vi "Profinet DCP Parsing.vi"(11 "Data in":string="\u0000\f)ÒîD\u0000\u001b\u001bI÷éˆ’þÿ\u0005\u0001\u0000\u0000\u0001k\u0000\u0000\u0000d\u0002\u0005\u0000\u001e\u0000\u0000\u0001\u0001\u0001\u0002\u0002\u0001\u0002\u0002\u0002\u0003\u0002\u0004\u0002\u0005\u0003=\u0005\u0001\u0005\u0002\u0005\u0003\u0005\u0004\u0005\u0005ÿÿ\u0002\u0001\u0000\u000b\u0000\u0000S7-400 CP\u0000\u0002\u0002\u0000\t\u0000\u0000pn-io-1\u0000\u0002\u0003\u0000\u0006\u0000\u0000\u0000*\u0002\u0001\u0002\u0004\u0000\u0004\u0000\u0000\u0002\u0000\u0001\u0002\u0000\u000e\u0000\u0001À¨dVÿÿÿ\u0000\u0000\u0000\u0000\u0000") -> (2 "PROFINET DCP Response":bool, 3 "Profinet Ident":T1)   [LabVIEW 2017]
uses:
  TypeDefs/control_packet_header_ethernet 2.ctl
  TypeDefs/Profinet Ident.ctl
panel:
  out "Device Role":u8[](array[numeric])
  out "Device ID":u8[](array[numeric])
  out "Device/Device Options":u8[](array[numeric])
  out "ethernet header":T2 {"Service ID and Type" format="%04x"; "Frame ID" format="%04x"; "destination MAC address"."?" format="%02x"; "destination MAC address"."?" format="%02x"; "destination MAC address"."?" format="%02x"; "destination MAC address"."?" format="%02x"; "destination MAC address"."?" format="%02x"; "destination MAC address"."?" format="%02x"; "source MAC address"."?" format="%02x"; "source MAC address"."?" format="%02x"; "source MAC address"."?" format="%02x"; "source MAC address"."?" format="%02x"; "source MAC address"."?" format="%02x"; "source MAC address"."?" format="%02x"; "length / type" format="%04x"}
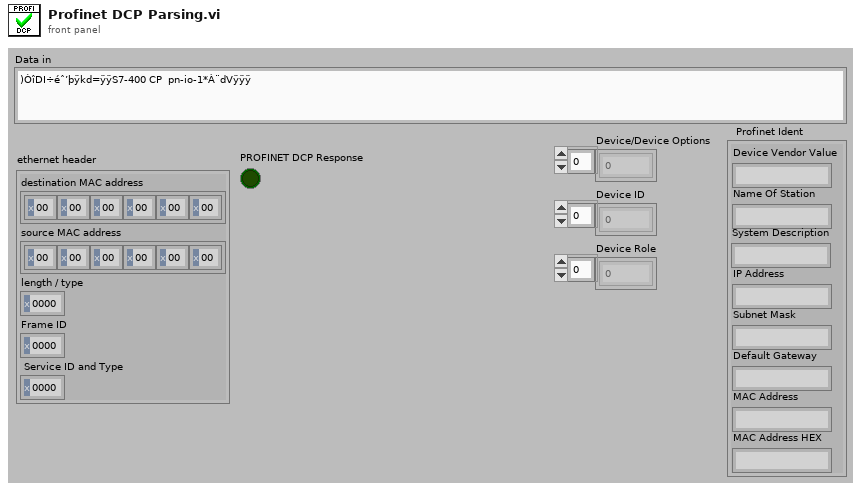
[diagram p1: front panel]
types:
  T1 = typedef "Profinet Ident.ctl" = cluster{"Device Vendor Value":string, "Name Of Station":string, "IP Address":string, "Subnet Mask":string, "Default Gateway":string, "MAC Address":string, "MAC Address HEX":string, "System Description ":string}
  T2 = typedef "control_packet_header_ethernet 2.ctl" = cluster{"destination MAC address":cluster{u8, u8, u8, u8, u8, u8}, "source MAC address":cluster{u8, u8, u8, u8, u8, u8}, "length / type":u16, "Frame ID":u16, " Service ID and Type":u16}
  T3 = enum16{"Device Type", "Device Vendor", "Name of Station", "Device ID", "Device Role", "IP Block", "Profinet Ident Values"}
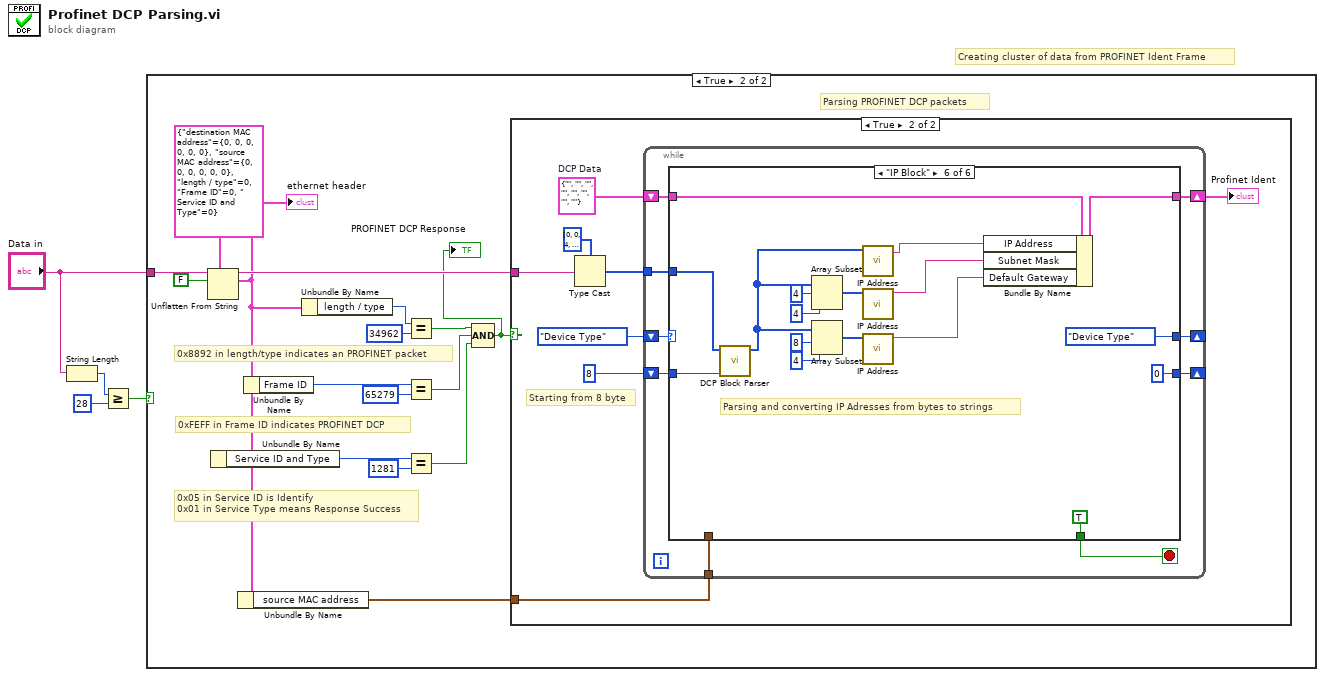
[diagram p0: block diagram]
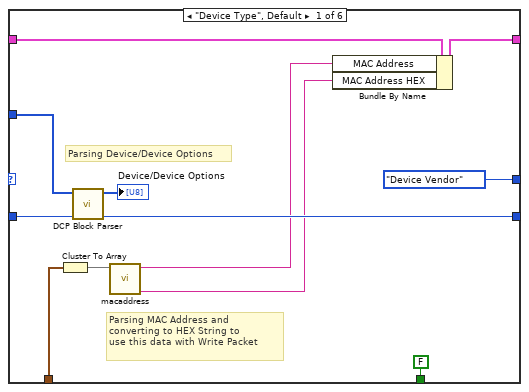
[diagram p4: hidden frame]
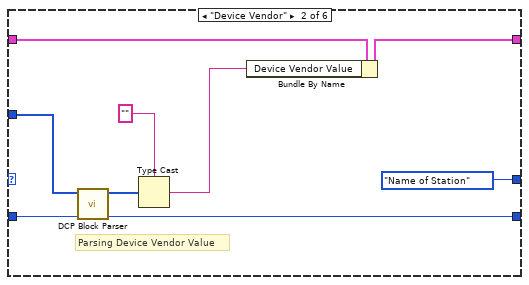
[diagram p5: hidden frame]
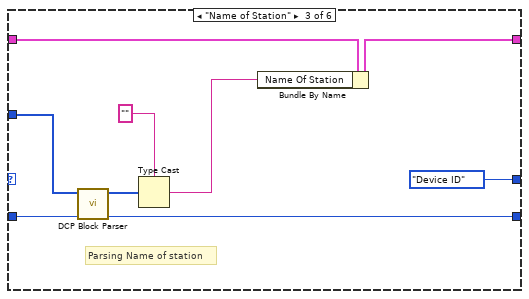
[diagram p6: hidden frame]
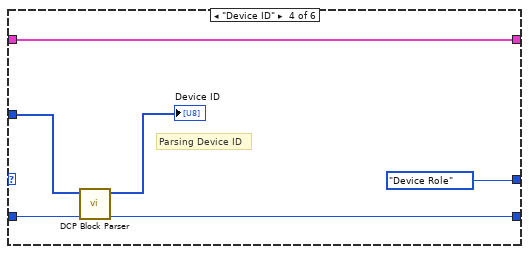
[diagram p7: hidden frame]
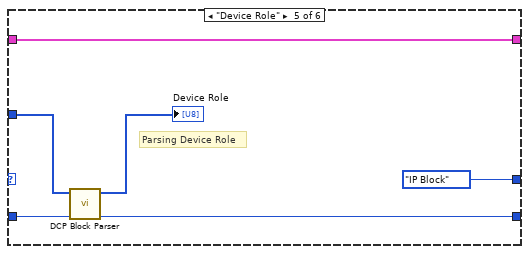
[diagram p8: hidden frame]
diagram:
  # "Creating cluster of data from PROFINET Ident Frame"
  n1 = String Length(string="Data in") -> (length=w3:i32)
  n2 = Greater Or Equal?(x=w3, y=28) -> (x >= y?=w1:bool)
  n3 = case shown="True" w1 {
    tunnel: "Data in" -> [_ w15]
    frame False {
    }
    frame True {
      # "0x05 in Service ID is Identify\n0x01 in Service Type means Response Success"
      # "0xFEFF in Frame ID indicates PROFINET DCP"
      # "Parsing PROFINET DCP packets"
      # "0x8892 in length/type indicates an PROFINET packet"
      n4 = Unflatten From String(type=T2 {"destination MAC address"={0, 0, 0, 0, 0, 0}, "source MAC address"={0, 0, 0, 0, 0, 0}, "length / type"=0, "Frame ID"=0, " Service ID and Type"=0} ("ethernet header"), binary string=w15, data includes array or string size? (T)=FALSE) -> (rest of the binary string=w16:string, value=w13:T2)  [unwired: 2 in, 1 out]
      "ethernet header" <- w13
      n5 = Unbundle By Name(w13) -> ("Service ID and Type"=w7:u16)
      n6 = Unbundle By Name(w13) -> ("source MAC address"=w14:cluster{u8, u8, u8, u8, u8, u8})
      n7 = Unbundle By Name(w13) -> ("Frame ID"=w12:u16)
      n8 = Unbundle By Name(w13) -> ("length / type"=w18:u16)
      n9 = Equal?(x=w18, y=u16 34962) -> (x = y?=w10:bool)
      n10 = Equal?(x=w12, y=u16 65279) -> (x = y?=w9:bool)
      n11 = Equal?(x=w7, y=u16 1281) -> (x = y?=w6:bool)
      n12 = Compound Arithmetic op=AND(w10, w9, w6) -> (w5:bool)
      "PROFINET DCP Response" <- w5
      n13 = case shown="True" w5 {
        tunnel: w16 -> [_ w28]
        tunnel: w14 -> [_ w27]
        frame False {
        }
        frame True {
          w22 = T1 {"Device Vendor Value"="", "Name Of Station"="", "IP Address"="", "Subnet Mask"="", "Default Gateway"="", "MAC Address"="", "MAC Address HEX"="", "System Description "=""}  # DCP Data
          # "Starting from 8 byte"
          n14 = Type Cast(type=u8[] [0, 0, 4, 0, 1, 0, 1, 0, 0, 0, 0, 0, 0, 0, 0, 0, 0, 0, 0, 0, 0, 0, 0, 0, 1, 0, 0, 0] ("Byte Array"), x=w28) -> (*(type *) &x=w25:u8[])
          n15 = while {
            tunnel: w25 -> [w37]
            shift-right: [w34] -> _
            shift-left: T3."Device Type" ("Enum") -> [w36]
            shift-right: [w33] -> _
            shift-left: 8 ("index") -> [w35]
            tunnel: w27 -> [w32]
            shift-right: [w30] -> w21
            shift-left: w22 -> [w29]
            stop <- w31 stop-if-true
            n16 = case shown="\"IP Block\"" w36 {
              tunnel: w37 -> [w49 w58 w67 w73 w79 w96]
              tunnel: w35 -> [w47 w57 w66 w71 w77 w95]
              tunnel: [T3."Device Vendor" ("Enum") T3."Name of Station" ("Enum") T3."Device ID" ("Enum") T3."Device Role" ("Enum") T3."IP Block" ("Enum") T3."Device Type" ("Enum")] -> w34
              tunnel: [w46 w56 w65 w70 w76 0 ("Block Last Byte")] -> w33
              tunnel: w32 -> [w44 _ _ _ _ _]
              tunnel: [FALSE _ _ _ _ TRUE] -> w31
              tunnel: w29 -> [w40 w52 w61 w68 w74 w86]
              tunnel: [w41 w51 w60 w68 w74 w85] -> w30
              frame "Device Type", Default {
                # "Parsing MAC Address and\nconverting to HEX String to\nuse this data with Write Packet"
                # "Parsing Device/Device Options"
                n17 = Cluster To Array(cluster=w44) -> (array=w45:u8[])
                n18 = call "DCP Block Parser.vi"("index"=w47, "Byte Array"=w49) -> ("Block Last Byte"=w46:i32, "Data"=→"Device/Device Options":u8[])  [unwired: 8 in]
                n19 = call "macaddress.vi"("source MAC address"=w45) -> ("MAC Address HEX"=w38:string, "MAC Address"=w39:string)  [unwired: 8 in]
                n20 = Bundle By Name(cluster=w40, "MAC Address"=w39, "MAC Address HEX"=w38) -> (w41:T1)
              }
              frame "Device Vendor" {
                # "Parsing Device Vendor Value"
                n21 = call "DCP Block Parser.vi"("index"=w57, "Byte Array"=w58) -> ("Block Last Byte"=w56:i32, "Data"=w55:u8[])  [unwired: 8 in]
                n22 = Type Cast(type="", x=w55) -> (*(type *) &x=w50:string)
                n23 = Bundle By Name(cluster=w52, "Device Vendor Value"=w50) -> (w51:T1)
              }
              frame "Name of Station" {
                # "Parsing Name of station"
                n24 = call "DCP Block Parser.vi"("index"=w66, "Byte Array"=w67) -> ("Block Last Byte"=w65:i32, "Data"=w63:u8[])  [unwired: 8 in]
                n25 = Type Cast(type="", x=w63) -> (*(type *) &x=w59:string)
                n26 = Bundle By Name(cluster=w61, "Name Of Station"=w59) -> (w60:T1)
              }
              frame "Device ID" {
                # "Parsing Device ID"
                n27 = call "DCP Block Parser.vi"("index"=w71, "Byte Array"=w73) -> ("Block Last Byte"=w70:i32, "Data"=→"Device ID":u8[])  [unwired: 8 in]
              }
              frame "Device Role" {
                # "Parsing Device Role"
                n28 = call "DCP Block Parser.vi"("index"=w77, "Byte Array"=w79) -> ("Block Last Byte"=w76:i32, "Data"=→"Device Role":u8[])  [unwired: 8 in]
              }
              frame "IP Block" {
                # "Parsing and converting IP Adresses from bytes to strings"
                n29 = call "DCP Block Parser.vi"("index"=w95, "Byte Array"=w96) -> ("Data"=w93:u8[])  [unwired: 8 in, 1 out]
                n30 = Array Subset(array=w93, index=4, length=4) -> (w91:u8[])
                n31 = Array Subset(array=w93, index=8, length=4) -> (w90:u8[])
                n32 = call "IP Address.vi"("Data"=w93) -> ("IP Address"=w84:string)  [unwired: 10 in]
                n33 = call "IP Address.vi"("Data"=w91) -> ("IP Address"=w83:string)  [unwired: 10 in]
                n34 = call "IP Address.vi"("Data"=w90) -> ("IP Address"=w82:string)  [unwired: 10 in]
                n35 = Bundle By Name(cluster=w86, "IP Address"=w84, "Subnet Mask"=w83, "Default Gateway"=w82) -> (w85:T1)
              }
            }
          }
          "Profinet Ident" <- w21
        }
      }
    }
  }
